vi "Load New Interpolation File.vi"(8 "error in (no error)":errorcluster, 10 "NewVal":path, 11 "Item Ref in":T1 format="%.0x") -> (0 "error out":errorcluster, 3 "Item Ref out":T1 format="%.0x")   [LabVIEW 2019, in "Profile Interpolation System Explorer.lvlib"]
uses:
  Profile Interpolation System Explorer.lvlib
  <vilib>/NI VeriStand/Custom Device API/Custom Device Item Ref.ctl
  Shared/Types/FG Action.ctl
  Types/Channel Sections.ctl
  <vilib>/NI VeriStand/Custom Device API/Custom Device Channel.ctl
  <vilib>/NI VeriStand/Custom Device API/Custom Device Channel Type.ctl
  Shared/SubVIs/Constants.vi
  <vilib>/NI VeriStand/Custom Device API/NI VeriStand - Get Item Property.vi
  <vilib>/NI VeriStand/Custom Device API/Get Item Property (Path).vi
  <vilib>/NI VeriStand/Custom Device API/Get Item Property (Boolean).vi
  <vilib>/NI VeriStand/Custom Device API/NI VeriStand - Set Item Property.vi
  <vilib>/NI VeriStand/Custom Device API/Set Item Property (Path).vi
  <vilib>/NI VeriStand/Custom Device API/Set Item Property (Boolean).vi
  <vilib>/NI VeriStand/Custom Device Tools/Custom Device Utility Library/NI VeriStand - Search for Item by GUID.vi
  <vilib>/NI VeriStand/Custom Device Tools/Custom Device Utility Library/Custom Device Utility Library.lvlib
  <vilib>/NI VeriStand/Custom Device API/Custom Device API.lvlib
  Shared/Profile Interpolation Shared.lvlib
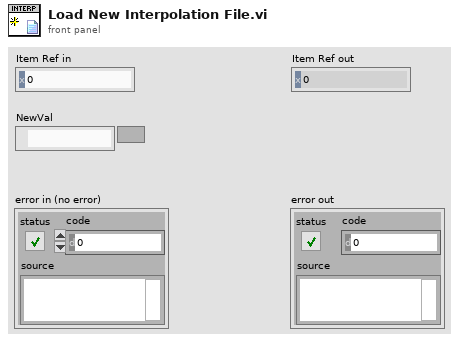
[diagram p1: front panel]
types:
  T1 = typedef "Custom Device API.lvlib/Custom Device Item Ref.ctl" = u64
  T2 = typedef "Profile Interpolation Shared.lvlib/FG Action.ctl" = enum8{"GET", "SET"}
  T3 = typedef "Profile Interpolation System Explorer.lvlib/Channel Sections.ctl" = enum16{"Initialize", "Table Section - Inputs", "Table Section - Outputs", "Status Section - Inputs", "Status Section - Outputs", "Exit"}
  T4 = typedef "Custom Device API.lvlib/Custom Device Channel.ctl" = cluster{"Type":T5, "Units":string, "Default Value":dbl, "Faultable":bool, "Scalable":bool}
  T5 = typedef "Custom Device API.lvlib/Custom Device Channel Type.ctl" = enum16{"Input", "Output"}
  T6 = typedef "Profile Interpolation Shared.lvlib/Interpolation Settings.ctl" = cluster{"Interpolation File":path, "Create Limit Channels?":bool}
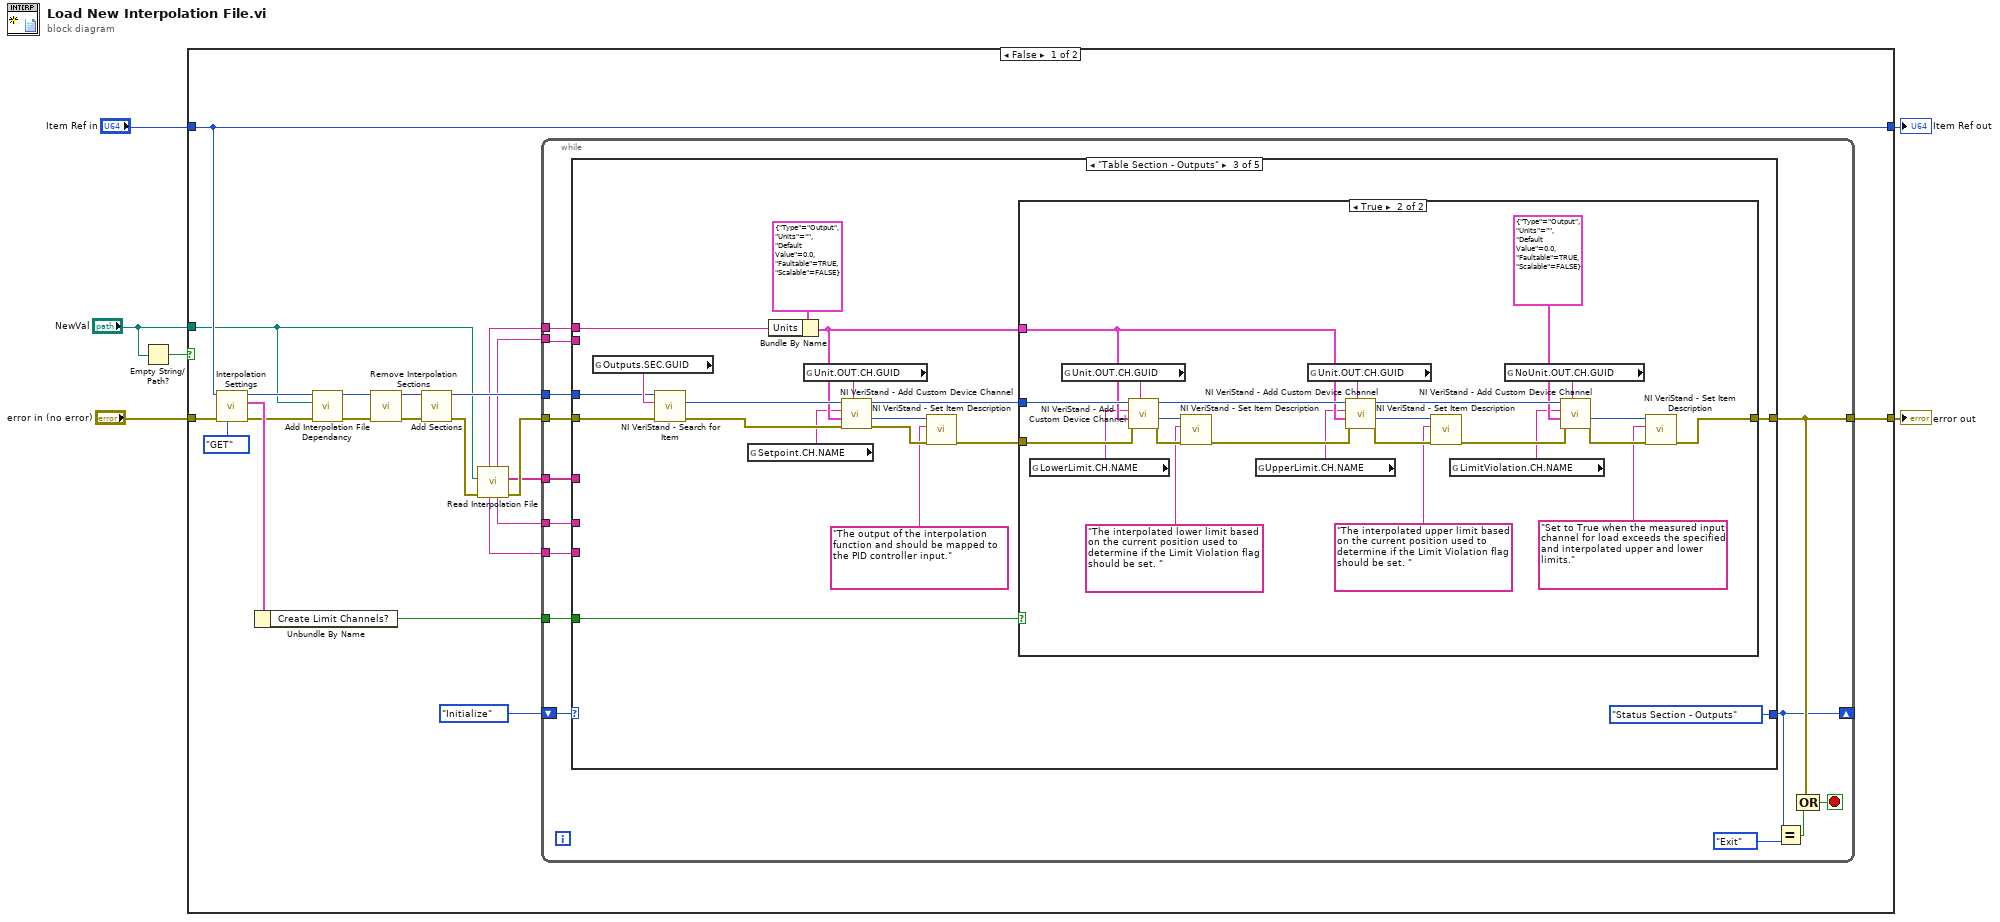
[diagram p0: block diagram]
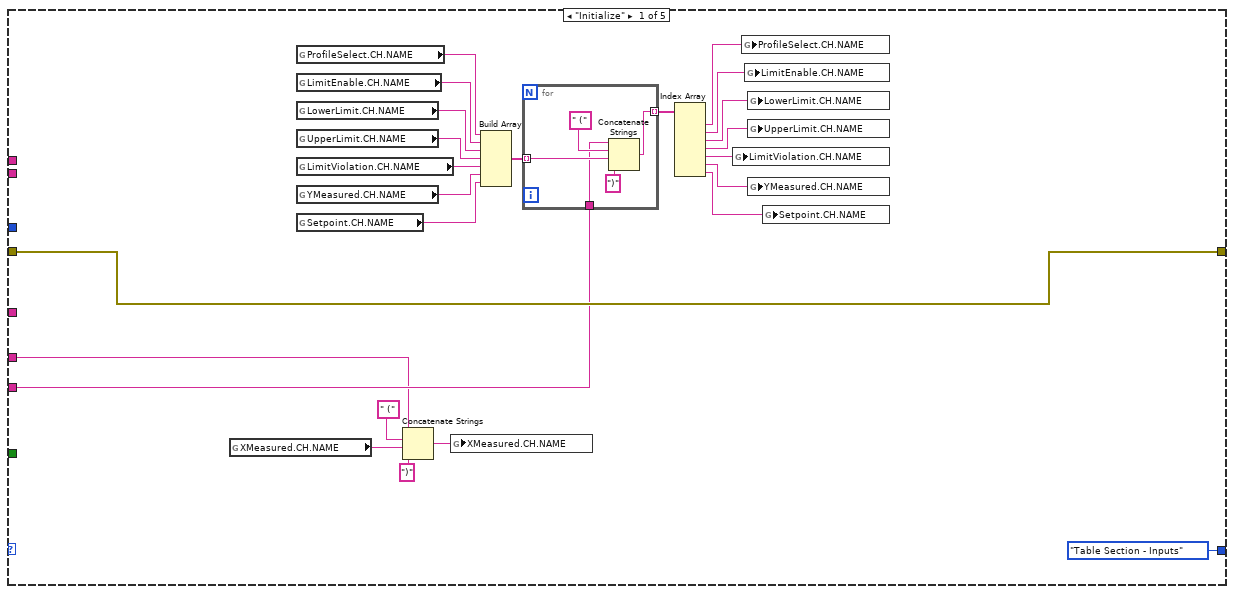
[diagram p2: hidden frame]
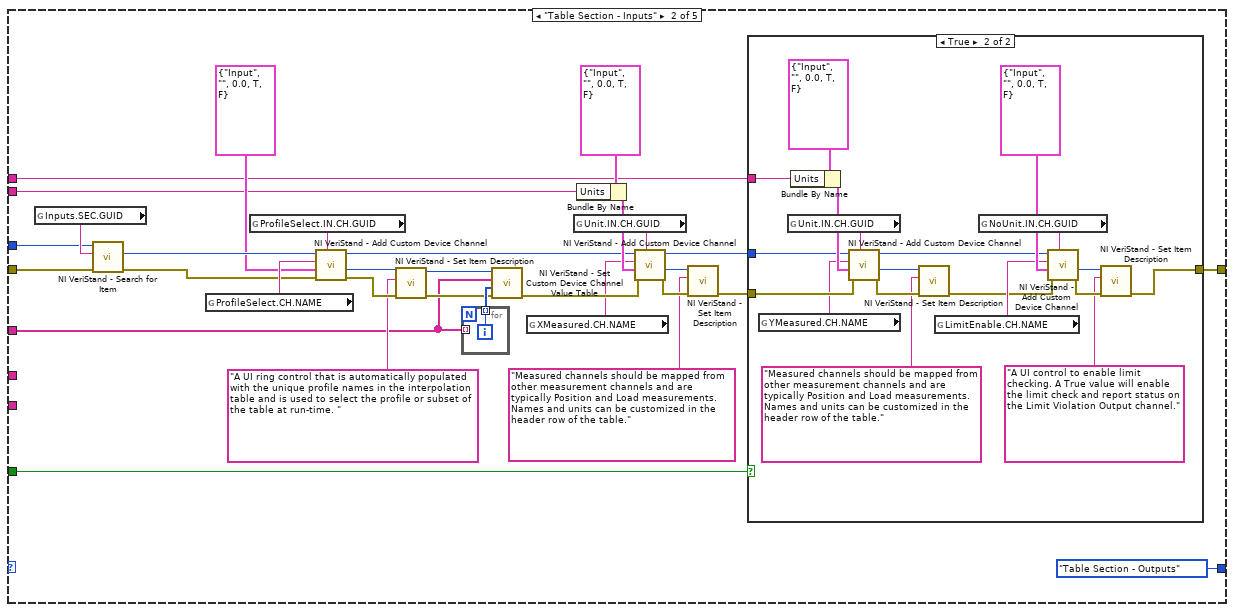
[diagram p3: hidden frame]
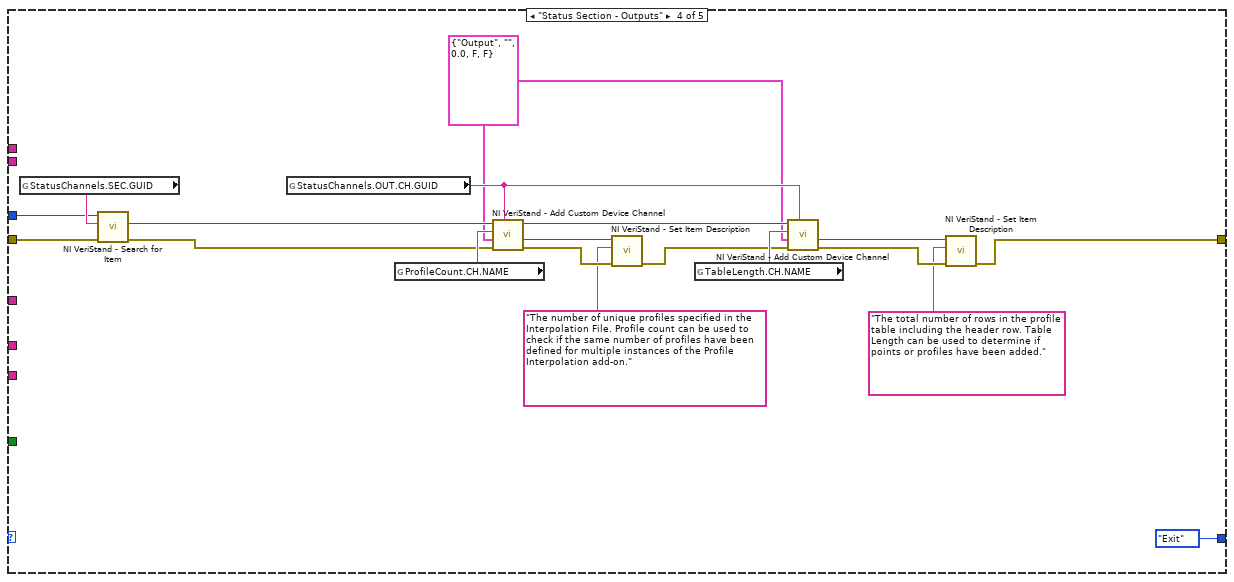
[diagram p6: hidden frame]
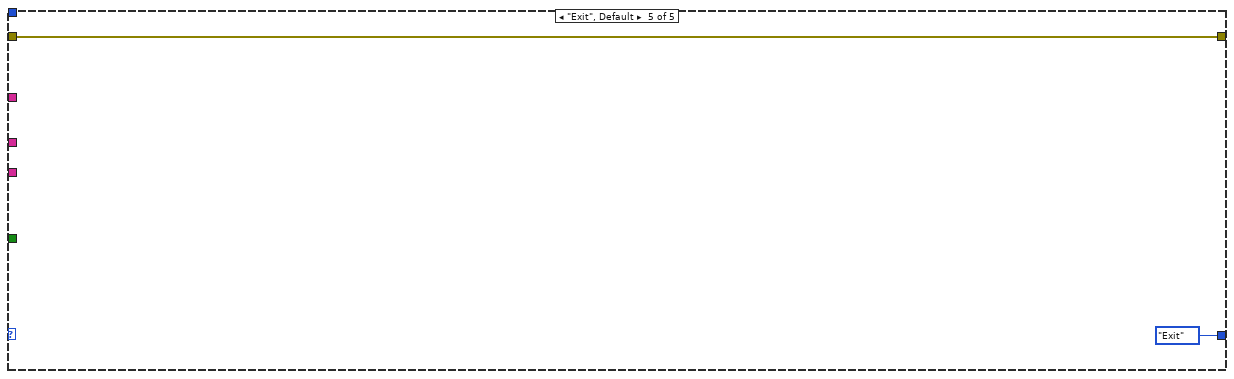
[diagram p7: hidden frame]
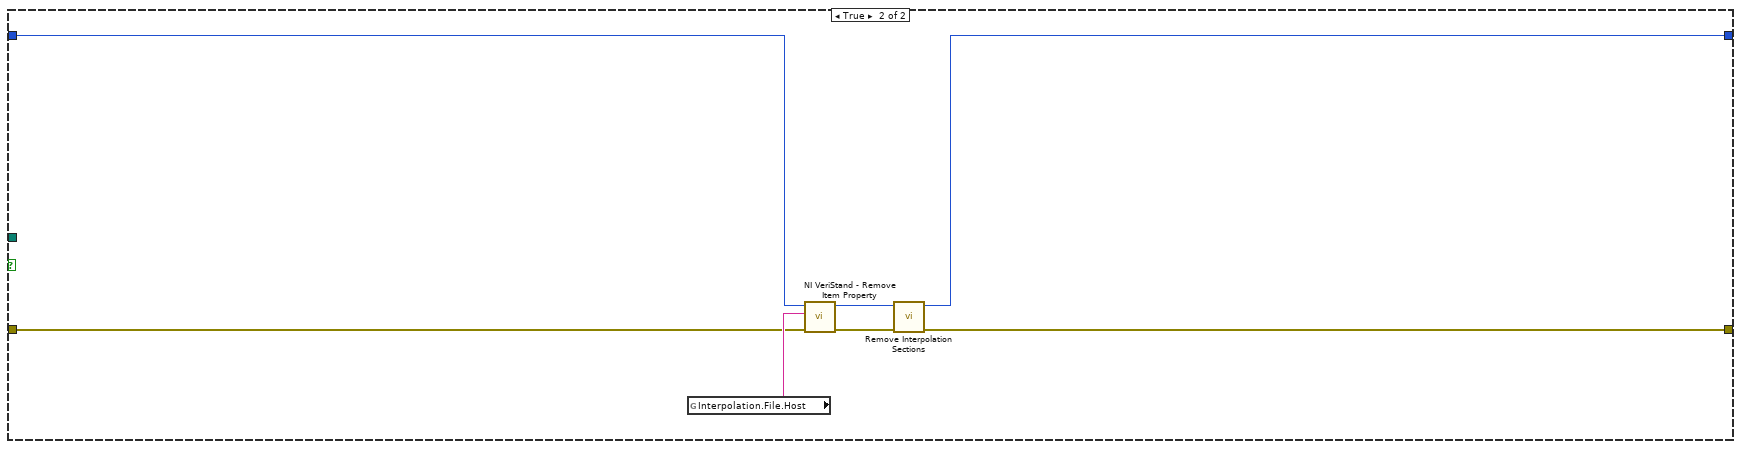
[diagram p8: hidden frame]
diagram:
  n1 = Empty String/Path?(string/path="NewVal") -> (empty?=w4:bool)
  n2 = case shown="False" w4 {
    tunnel: "NewVal" -> [w12 _]
    tunnel: "error in (no error)" -> [w19 w191]
    tunnel: [w27 w194] -> w6
    tunnel: [w20 w188] -> w5
    tunnel: "Item Ref in" -> [w20 w189]
    frame False {
      n3 = call "Interpolation Settings.vi"("Action"=FG_Action."GET", "error in (no error)"=w19, "Item Ref"=w20) -> ("error out"=w17:errorcluster, "Interpolation Settings out"=w21:T6, "Item Ref out"=w18:T1)  [unwired: 6 in]
      n4 = Unbundle By Name(w21) -> ("Create Limit Channels?"=w23:bool)
      n5 = call "Add Interpolation File Dependancy.vi"("error in (no error)"=w17, "Path"=w12, "Item Ref in"=w18) -> ("error out"=w15:errorcluster, "Item Ref out"=w16:T1)  [unwired: 7 in]
      n6 = call "Remove Interpolation Sections.vi"("error in (no error)"=w15, "Item Ref in"=w16) -> ("error out"=w28:errorcluster, "Item Ref out"=w25:T1)  [unwired: 8 in]
      n7 = call "Add Sections.vi"("error in (no error)"=w28, "Item Ref in"=w25) -> ("error out"=w14:errorcluster, "Item Ref out"=w22:T1)  [unwired: 8 in]
      n8 = call "Read Interpolation File.vi"("error in"=w14, "file path (dialog if empty)"=w12) -> ("error out"=w13:errorcluster, "Profiles"=w7:string[], "xName"=w9:string, "xUnit"=w10:string, "yName"=w8:string, "yUnit"=w11:string)  [unwired: 2 in, 2 out]
      n9 = while {
        tunnel: [w41] -> w27
        tunnel: w13 -> [w42]
        shift-right: [w37] -> _
        shift-left: Channel_Sections."Initialize" -> [w39]
        tunnel: w22 -> [w38]
        tunnel: w23 -> [w34]
        tunnel: w11 -> [w30]
        tunnel: w10 -> [w31]
        tunnel: w9 -> [w33]
        tunnel: w8 -> [w32]
        tunnel: w7 -> [w29]
        stop <- w40 stop-if-true
        n10 = case shown="\"Table Section - Outputs\"" w39 {
          tunnel: [w53 w83 w128 w175 w187] -> w41
          tunnel: w42 -> [w53 w81 w140 w177 w187]
          tunnel: [Channel_Sections."Table Section - Inputs" Channel_Sections."Table Section - Outputs" Channel_Sections."Status Section - Outputs" Channel_Sections."Exit" Channel_Sections."Exit"] -> w37
          tunnel: w38 -> [_ w82 w138 w167 _]
          tunnel: w34 -> [_ w80 w127 _ _]
          tunnel: w33 -> [w49 _ _ _ _]
          tunnel: w32 -> [w52 _ _ _ _]
          tunnel: w31 -> [_ w77 _ _ _]
          tunnel: w30 -> [_ w76 w125 _ _]
          tunnel: w29 -> [_ w75 _ _ _]
          frame "Initialize" {
            n11 = global read "Constants.vi" "XMeasured.CH.NAME"() -> (w48:string)
            n12 = global read "Constants.vi" "ProfileSelect.CH.NAME"() -> (w65:string)
            n13 = global read "Constants.vi" "LimitEnable.CH.NAME"() -> (w64:string)
            n14 = global read "Constants.vi" "LowerLimit.CH.NAME"() -> (w63:string)
            n15 = global read "Constants.vi" "UpperLimit.CH.NAME"() -> (w62:string)
            n16 = global read "Constants.vi" "LimitViolation.CH.NAME"() -> (w61:string)
            n17 = global read "Constants.vi" "YMeasured.CH.NAME"() -> (w44:string)
            n18 = global read "Constants.vi" "Setpoint.CH.NAME"() -> (w43:string)
            n19 = Concatenate Strings(w49, " (" ("string"), w48, ")" ("string")) -> (w47:string)
            n20 = global write "Constants.vi" "XMeasured.CH.NAME"(w47) -> ()
            n21 = Build Array(w65, w64, w63, w62, w61, w44, w43) -> (w60:string[])
            n22 = for {
              tunnel: w60 -> [w70] mode=indexing
              tunnel: [w68] -> w54 mode=indexing
              tunnel: w52 -> [w67]
              n23 = Concatenate Strings(w67, " (" ("string"), w70, ")" ("string")) -> (w68:string)
            }
            n24 = Index Array(array=w54) -> (element #1=w59:string, element #2=w58:string, element #3=w57:string, element #4=w56:string, element #5=w55:string, element #6=w46:string, element #7=w45:string)  [unwired: 7 in]
            n25 = global write "Constants.vi" "LimitViolation.CH.NAME"(w55) -> ()
            n26 = global write "Constants.vi" "ProfileSelect.CH.NAME"(w59) -> ()
            n27 = global write "Constants.vi" "LimitEnable.CH.NAME"(w58) -> ()
            n28 = global write "Constants.vi" "LowerLimit.CH.NAME"(w57) -> ()
            n29 = global write "Constants.vi" "UpperLimit.CH.NAME"(w56) -> ()
            n30 = global write "Constants.vi" "YMeasured.CH.NAME"(w46) -> ()
            n31 = global write "Constants.vi" "Setpoint.CH.NAME"(w45) -> ()
          }
          frame "Table Section - Inputs" {
            n32 = global read "Constants.vi" "Inputs.SEC.GUID"() -> (w100:string)
            n33 = call-poly <vilib>:"NI VeriStand - Search for Item.vi"("error in"=w81, "Item GUID"=w100, "Section Ref in"=w82) -> ("error out"=w73:errorcluster, "Item Ref"=w96:T1)  [unwired: 5 in, 2 out]
            n34 = global read "Constants.vi" "ProfileSelect.CH.NAME"() -> (w95:string)
            n35 = global read "Constants.vi" "ProfileSelect.IN.CH.GUID"() -> (w99:string)
            n36 = call <vilib>:"NI VeriStand - Add Custom Device Channel.vi"("GUID (Default Channel)"=w99, "error in (no error)"=w73, "Channel"=T4 {"Type"=enum."Input", "Units"="", "Default Value"=0.0, "Faultable"=TRUE, "Scalable"=FALSE}, "Channel Name"=w95, "Parent Ref in"=w96) -> ("error out"=w88:errorcluster, "Channel Ref"=w87:T1, "Parent Ref out"=w72:T1)  [unwired: 3 in, 1 out]
            n37 = call <vilib>:"NI VeriStand - Set Item Description.vi"("error in (no error)"=w88, "Description"="A UI ring control that is automatically populated with the unique profile names in the interpolation table and is used to select the profile or subset of the table at run-time. " ("String"), "Item Ref in"=w87) -> ("error out"=w85:errorcluster, "Item Ref out"=w86:T1)  [unwired: 7 out]
            n38 = for {
              tunnel: [w123] -> w101 mode=indexing
              tunnel: w75 -> [_] mode=indexing
              i -> [w123]
            }
            n39 = call <vilib>:"NI VeriStand - Set Custom Device Channel Value Table.vi"("error in (no error)"=w85, "Values"=w101, "Names"=w75, "Channel Ref in"=w86) -> ("error out"=w98:errorcluster)  [unwired: 6 in, 1 out]
            n40 = global read "Constants.vi" "XMeasured.CH.NAME"() -> (w74:string)
            n41 = global read "Constants.vi" "Unit.IN.CH.GUID"() -> (w97:string)
            n42 = Bundle By Name(cluster=T4 {"Type"=enum."Input", "Units"="", "Default Value"=0.0, "Faultable"=TRUE, "Scalable"=FALSE} ("Channel"), "Units"=w77) -> (w102:T4)
            n43 = call <vilib>:"NI VeriStand - Add Custom Device Channel.vi"("GUID (Default Channel)"=w97, "error in (no error)"=w98, "Channel"=w102, "Channel Name"=w74, "Parent Ref in"=w72) -> ("error out"=w94:errorcluster, "Channel Ref"=w93:T1, "Parent Ref out"=w78:T1)  [unwired: 3 in, 1 out]
            n44 = call <vilib>:"NI VeriStand - Set Item Description.vi"("error in (no error)"=w94, "Description"="Measured channels should be mapped from other measurement channels and are typically Position and Load measurements. Names and units can be customized in the header row of the table." ("String"), "Item Ref in"=w93) -> ("error out"=w79:errorcluster)  [unwired: 8 out]
            n45 = case shown="True" w80 {
              tunnel: w79 -> [w103 w107]
              tunnel: w78 -> [_ w109]
              tunnel: [w103 w116] -> w83
              tunnel: w76 -> [_ w108]
              frame False {
              }
              frame True {
                n46 = global read "Constants.vi" "YMeasured.CH.NAME"() -> (w104:string)
                n47 = global read "Constants.vi" "Unit.IN.CH.GUID"() -> (w114:string)
                n48 = Bundle By Name(cluster=T4 {"Type"=enum."Input", "Units"="", "Default Value"=0.0, "Faultable"=TRUE, "Scalable"=FALSE} ("Channel"), "Units"=w108) -> (w115:T4)
                n49 = call <vilib>:"NI VeriStand - Add Custom Device Channel.vi"("GUID (Default Channel)"=w114, "error in (no error)"=w107, "Channel"=w115, "Channel Name"=w104, "Parent Ref in"=w109) -> ("error out"=w113:errorcluster, "Channel Ref"=w112:T1, "Parent Ref out"=w106:T1)  [unwired: 3 in, 1 out]
                n50 = call <vilib>:"NI VeriStand - Set Item Description.vi"("error in (no error)"=w113, "Description"="Measured channels should be mapped from other measurement channels and are typically Position and Load measurements. Names and units can be customized in the header row of the table." ("String"), "Item Ref in"=w112) -> ("error out"=w105:errorcluster)  [unwired: 8 out]
                n51 = global read "Constants.vi" "LimitEnable.CH.NAME"() -> (w117:string)
                n52 = global read "Constants.vi" "NoUnit.IN.CH.GUID"() -> (w120:string)
                n53 = call <vilib>:"NI VeriStand - Add Custom Device Channel.vi"("GUID (Default Channel)"=w120, "error in (no error)"=w105, "Channel"=T4 {"Type"=enum."Input", "Units"="", "Default Value"=0.0, "Faultable"=TRUE, "Scalable"=FALSE}, "Channel Name"=w117, "Parent Ref in"=w106) -> ("error out"=w121:errorcluster, "Channel Ref"=w122:T1)  [unwired: 3 in, 2 out]
                n54 = call <vilib>:"NI VeriStand - Set Item Description.vi"("error in (no error)"=w121, "Description"="A UI control to enable limit checking. A True value will enable the limit check and report status on the Limit Violation Output channel." ("String"), "Item Ref in"=w122) -> ("error out"=w116:errorcluster)  [unwired: 8 out]
              }
            }
          }
          frame "Table Section - Outputs" {
            n55 = global read "Constants.vi" "Outputs.SEC.GUID"() -> (w141:string)
            n56 = call-poly <vilib>:"NI VeriStand - Search for Item.vi"("error in"=w140, "Item GUID"=w141, "Section Ref in"=w138) -> ("error out"=w126:errorcluster, "Item Ref"=w130:T1)  [unwired: 5 in, 2 out]
            n57 = global read "Constants.vi" "Setpoint.CH.NAME"() -> (w124:string)
            n58 = Bundle By Name(cluster=T4 {"Type"=enum."Output", "Units"="", "Default Value"=0.0, "Faultable"=TRUE, "Scalable"=FALSE} ("Channel"), "Units"=w125) -> (w129:T4)
            n59 = global read "Constants.vi" "Unit.OUT.CH.GUID"() -> (w137:string)
            n60 = call <vilib>:"NI VeriStand - Add Custom Device Channel.vi"("GUID (Default Channel)"=w137, "error in (no error)"=w126, "Channel"=w129, "Channel Name"=w124, "Parent Ref in"=w130) -> ("error out"=w136:errorcluster, "Channel Ref"=w135:T1, "Parent Ref out"=w132:T1)  [unwired: 3 in, 1 out]
            n61 = call <vilib>:"NI VeriStand - Set Item Description.vi"("error in (no error)"=w136, "Description"="The output of the interpolation function and should be mapped to the PID controller input." ("String"), "Item Ref in"=w135) -> ("error out"=w131:errorcluster)  [unwired: 8 out]
            n62 = case shown="True" w127 {
              tunnel: w132 -> [_ w156]
              tunnel: w131 -> [w142 w155]
              tunnel: w129 -> [_ w154]
              tunnel: [w142 w147] -> w128
              frame False {
              }
              frame True {
                n63 = global read "Constants.vi" "LowerLimit.CH.NAME"() -> (w144:string)
                n64 = global read "Constants.vi" "Unit.OUT.CH.GUID"() -> (w165:string)
                n65 = call <vilib>:"NI VeriStand - Add Custom Device Channel.vi"("GUID (Default Channel)"=w165, "error in (no error)"=w155, "Channel"=w154, "Channel Name"=w144, "Parent Ref in"=w156) -> ("error out"=w163:errorcluster, "Channel Ref"=w160:T1, "Parent Ref out"=w161:T1)  [unwired: 3 in, 1 out]
                n66 = call <vilib>:"NI VeriStand - Set Item Description.vi"("error in (no error)"=w163, "Description"="The interpolated lower limit based on the current position used to determine if the Limit Violation flag should be set. " ("String"), "Item Ref in"=w160) -> ("error out"=w162:errorcluster)  [unwired: 8 out]
                n67 = global read "Constants.vi" "UpperLimit.CH.NAME"() -> (w143:string)
                n68 = global read "Constants.vi" "Unit.OUT.CH.GUID"() -> (w166:string)
                n69 = call <vilib>:"NI VeriStand - Add Custom Device Channel.vi"("GUID (Default Channel)"=w166, "error in (no error)"=w162, "Channel"=w154, "Channel Name"=w143, "Parent Ref in"=w161) -> ("error out"=w164:errorcluster, "Channel Ref"=w159:T1, "Parent Ref out"=w149:T1)  [unwired: 3 in, 1 out]
                n70 = call <vilib>:"NI VeriStand - Set Item Description.vi"("error in (no error)"=w164, "Description"="The interpolated upper limit based on the current position used to determine if the Limit Violation flag should be set. " ("String"), "Item Ref in"=w159) -> ("error out"=w148:errorcluster)  [unwired: 8 out]
                n71 = global read "Constants.vi" "LimitViolation.CH.NAME"() -> (w145:string)
                n72 = global read "Constants.vi" "NoUnit.OUT.CH.GUID"() -> (w153:string)
                n73 = call <vilib>:"NI VeriStand - Add Custom Device Channel.vi"("GUID (Default Channel)"=w153, "error in (no error)"=w148, "Channel"=T4 {"Type"=enum."Output", "Units"="", "Default Value"=0.0, "Faultable"=TRUE, "Scalable"=FALSE}, "Channel Name"=w145, "Parent Ref in"=w149) -> ("error out"=w152:errorcluster, "Channel Ref"=w151:T1)  [unwired: 3 in, 2 out]
                n74 = call <vilib>:"NI VeriStand - Set Item Description.vi"("error in (no error)"=w152, "Description"="Set to True when the measured input channel for load exceeds the specified and interpolated upper and lower limits." ("String"), "Item Ref in"=w151) -> ("error out"=w147:errorcluster)  [unwired: 8 out]
              }
            }
          }
          frame "Status Section - Outputs" {
            w178 = T4 {"Type"=enum."Output", "Units"="", "Default Value"=0.0, "Faultable"=FALSE, "Scalable"=FALSE} ("Channel")
            n75 = global read "Constants.vi" "StatusChannels.SEC.GUID"() -> (w185:string)
            n76 = call-poly <vilib>:"NI VeriStand - Search for Item.vi"("error in"=w177, "Item GUID"=w185, "Section Ref in"=w167) -> ("error out"=w179:errorcluster, "Item Ref"=w181:T1)  [unwired: 5 in, 2 out]
            n77 = global read "Constants.vi" "StatusChannels.OUT.CH.GUID"() -> (w184:string)
            n78 = global read "Constants.vi" "ProfileCount.CH.NAME"() -> (w183:string)
            n79 = call <vilib>:"NI VeriStand - Add Custom Device Channel.vi"("GUID (Default Channel)"=w184, "error in (no error)"=w179, "Channel"=w178, "Channel Name"=w183, "Parent Ref in"=w181) -> ("error out"=w171:errorcluster, "Channel Ref"=w172:T1, "Parent Ref out"=w182:T1)  [unwired: 3 in, 1 out]
            n80 = call <vilib>:"NI VeriStand - Set Item Description.vi"("error in (no error)"=w171, "Description"="The number of unique profiles specified in the Interpolation File. Profile count can be used to check if the same number of profiles have been defined for multiple instances of the Profile Interpolation add-on." ("Name"), "Item Ref in"=w172) -> ("error out"=w170:errorcluster)  [unwired: 8 out]
            n81 = global read "Constants.vi" "TableLength.CH.NAME"() -> (w180:string)
            n82 = call <vilib>:"NI VeriStand - Add Custom Device Channel.vi"("GUID (Default Channel)"=w184, "error in (no error)"=w170, "Channel"=w178, "Channel Name"=w180, "Parent Ref in"=w182) -> ("error out"=w176:errorcluster, "Channel Ref"=w174:T1)  [unwired: 3 in, 2 out]
            n83 = call <vilib>:"NI VeriStand - Set Item Description.vi"("error in (no error)"=w176, "Description"="The total number of rows in the profile table including the header row. Table Length can be used to determine if points or profiles have been added." ("String"), "Item Ref in"=w174) -> ("error out"=w175:errorcluster)  [unwired: 8 out]
          }
          frame "Exit", Default {
          }
        }
        n84 = Equal?(x=w37, y=Channel_Sections."Exit") -> (x = y?=w35:bool)
        n85 = Compound Arithmetic op=OR(w41, w35) -> (w40:bool)
      }
    }
    frame True {
      n86 = global read "Constants.vi" "Interpolation.File.Host"() -> (w193:string)
      n87 = call <vilib>:"NI VeriStand - Remove Item Property.vi"("error in (no error)"=w191, "Property Name"=w193, "Item Ref in"=w189) -> ("error out"=w190:errorcluster, "Item Ref out"=w192:T1)  [unwired: 6 in, 1 out]
      n88 = call "Remove Interpolation Sections.vi"("error in (no error)"=w190, "Item Ref in"=w192) -> ("error out"=w194:errorcluster, "Item Ref out"=w188:T1)  [unwired: 8 in]
    }
  }
  "error out" <- w6
  "Item Ref out" <- w5
